vi "Configak.vi"() -> ()   [LabVIEW 2020]
uses:
  Global_Variable/A131258.vi
  Database/Global1.vi
  Global_Variable/Global.vi
  <vilib>/Utility/config.llb/NI_LVConfig.lvlib
panel:
  in  "系数":bool
  in  "产品型号":string(combo)
  in  "删除":bool
  in  "确定":bool
  in  "添加":bool
  in  "退出":bool
  in  "更新":bool
  in  "选项卡控件":enum32{"产品参数", "系统参数"}(tab)
  in  "复选框":bool
  in  "判定框范围":string[][](table)=[["°"], ["N"], ["°"], ["N"], ["°"], ["N"], ["°"], ["N"]]
  in  "工位坐标轴参数":string[][](table)=[["°"], ["N"], ["°"], ["N"], ["mm"], ["N"], ["mm"], ["N"]]
  in  "结果判定参数":string[][](table)=[["N"], ["N"], ["N"], ["N"], ["N"], ["N"], ["N"], ["N"], ["N"]]
  in  "工位滤波":T1
  in  "系统参数设置":string[][](table)=[[""], [""], [""], [""]]
  # "磨合台"
types:
  T1 = cluster{"左滤波":bool, "系数1":dbl, "右滤波":bool, "系数 2":dbl}
  T2 = enum8{"Enabled", "Disabled", "Disabled and Grayed Out"}
  T3 = typedef "NI_LVConfig.lvlib/Config Data RefNum.ctl" = refnum<k1>
  T4 = cluster{"用户编号":string, "用户名":string, "用户密码(密文)":string, "用户权限":string}
  T5 = cluster{"[0]":cluster{dbl, dbl}, "[1]":cluster{dbl, dbl}, "[2]":cluster{dbl, dbl}, "[3]":cluster{dbl, dbl}, "[4]":cluster{dbl, dbl}, "[5]":cluster{dbl, dbl}, "[6]":cluster{dbl, dbl}, "[7]":cluster{dbl, dbl}, "[8]":cluster{dbl, dbl}, "[9]":cluster{dbl, dbl}, "[10]":cluster{dbl, dbl}}
  T6 = cluster{"[0]":cluster{string, dbl, dbl}, "[1]":cluster{string, dbl, dbl}, "[2]":cluster{string, dbl, dbl}, "[3]":cluster{string, dbl, dbl}}
  T7 = cluster{"[0]":cluster{string, dbl, dbl}, "[1]":cluster{string, dbl, dbl}, "[2]":cluster{string, dbl, dbl}, "[3]":cluster{string, dbl, dbl}, "[4]":cluster{string, dbl, dbl}, "[5]":cluster{string, dbl, dbl}, "[6]":cluster{string, dbl, dbl}, "[7]":cluster{string, dbl, dbl}, "[8]":cluster{string, dbl, dbl}, "[9]":cluster{string, dbl, dbl}}
  T8 = cluster{"正向判定X值":cluster{"单位":string, "下限":dbl, "上限":dbl}, "正向判定Y值":cluster{"单位":string, "下限":dbl, "上限":dbl}, "逆向判定X值":cluster{"单位":string, "下限":dbl, "上限":dbl}, "逆向判定Y值":cluster{"单位":string, "下限":dbl, "上限":dbl}}
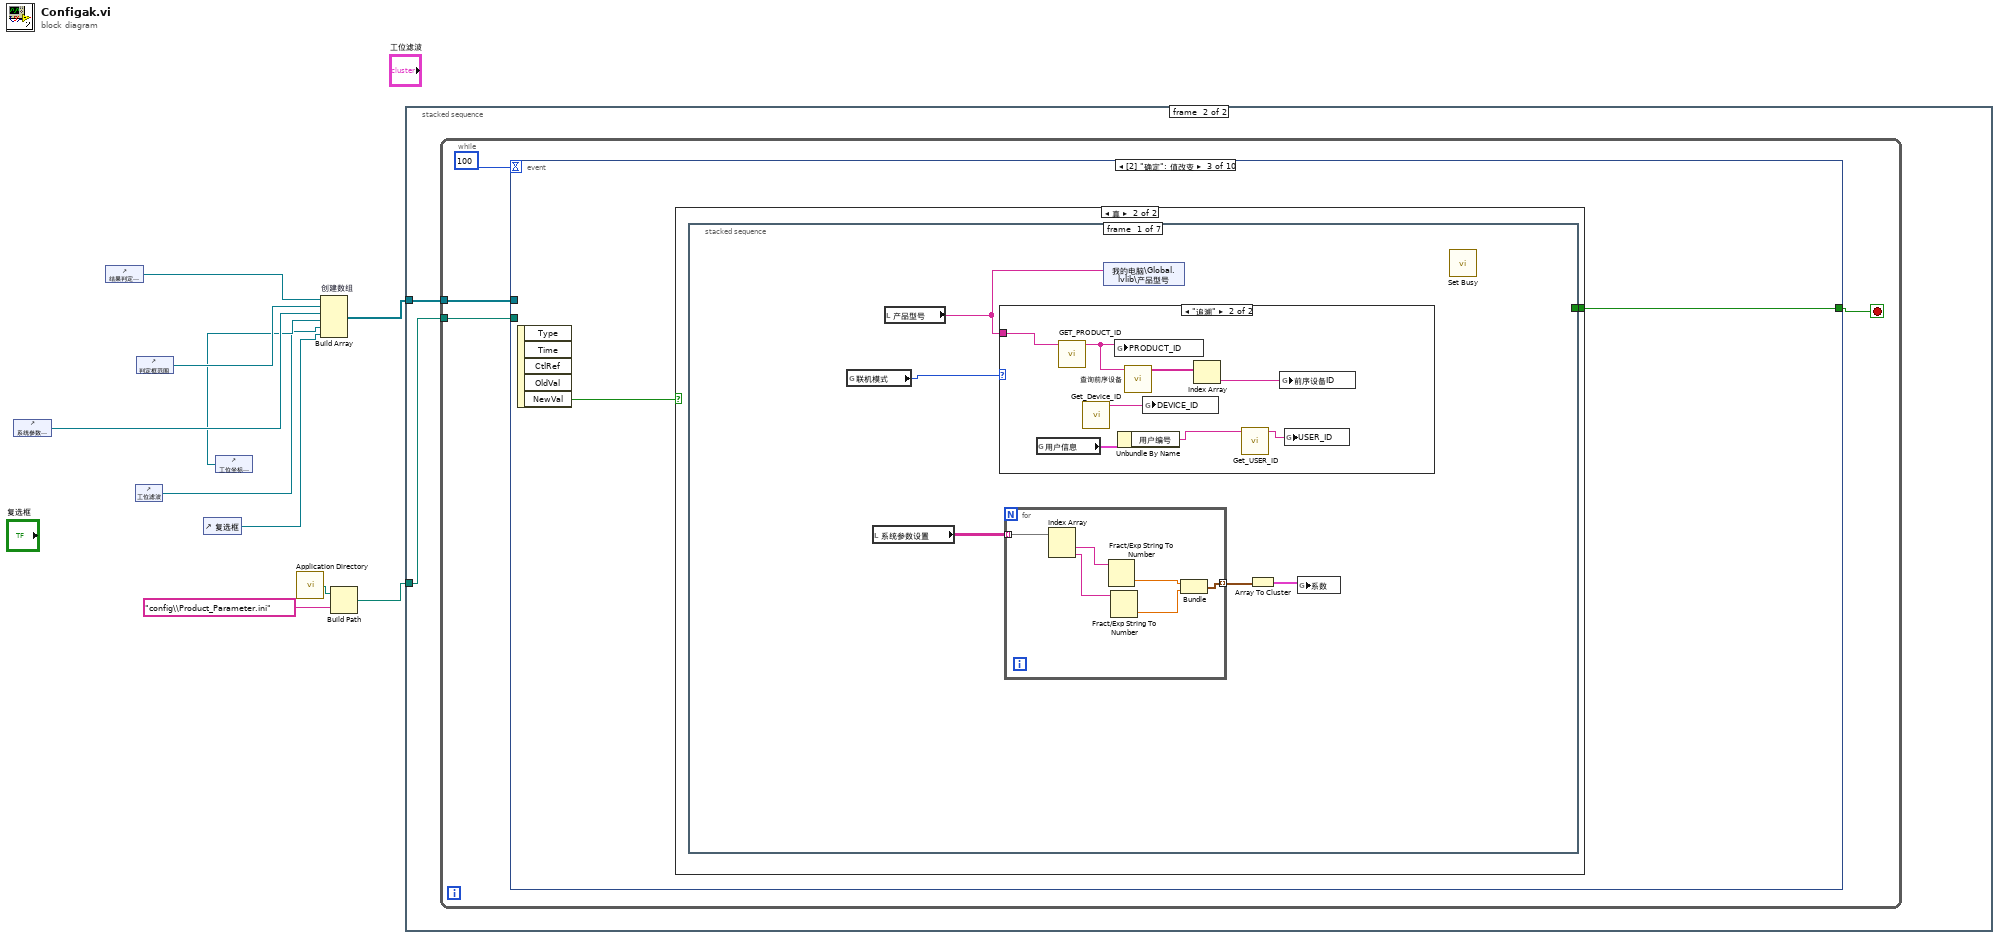
[diagram p0: block diagram]
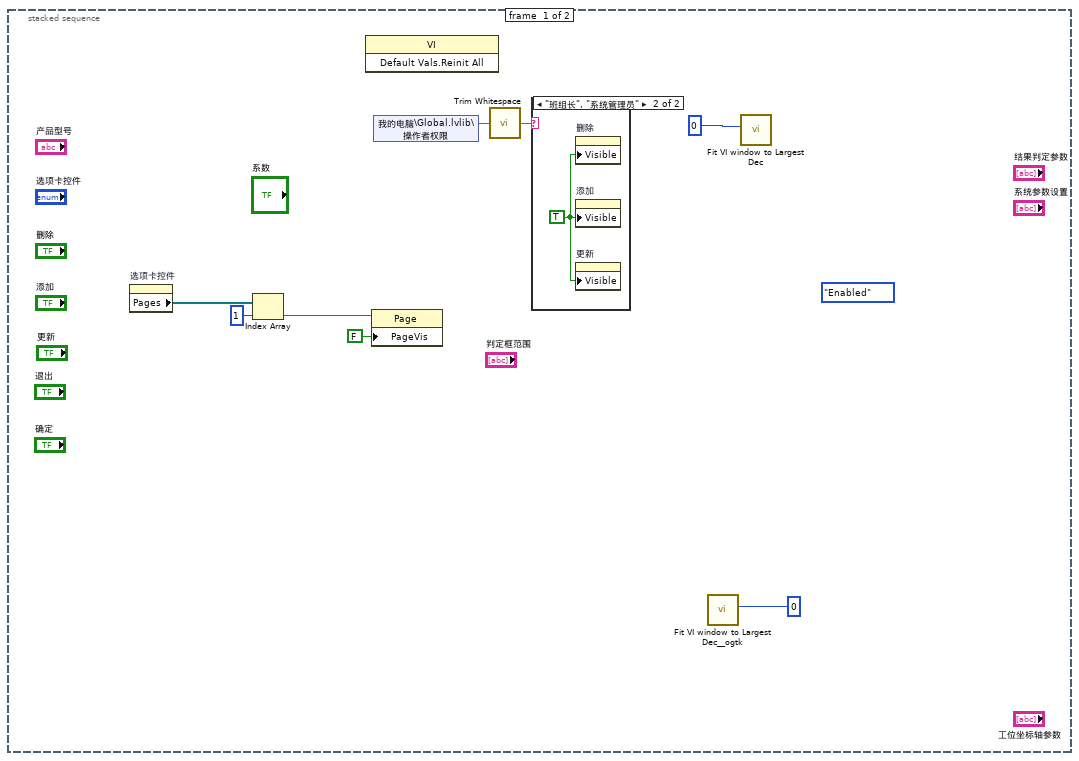
[diagram p2: hidden frame]
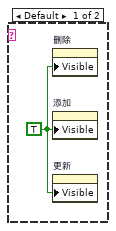
[diagram p3: hidden frame]
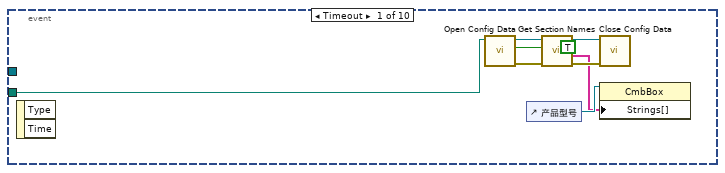
[diagram p4: hidden frame]
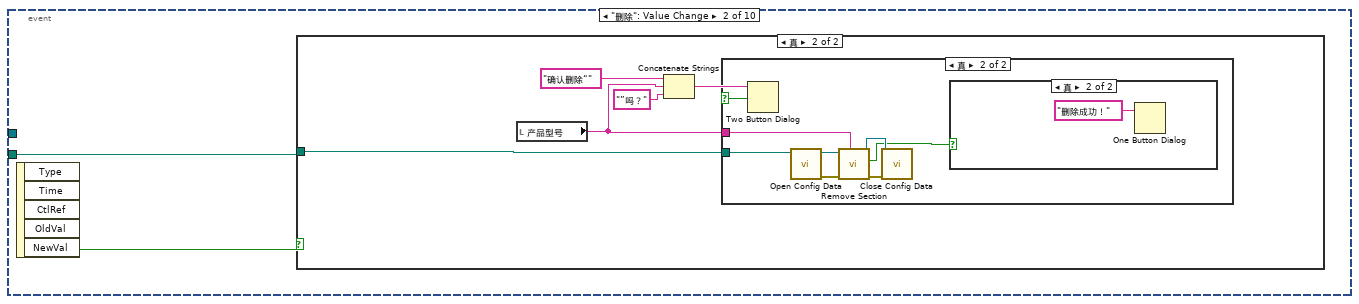
[diagram p5: hidden frame]
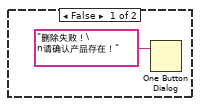
[diagram p8: hidden frame]
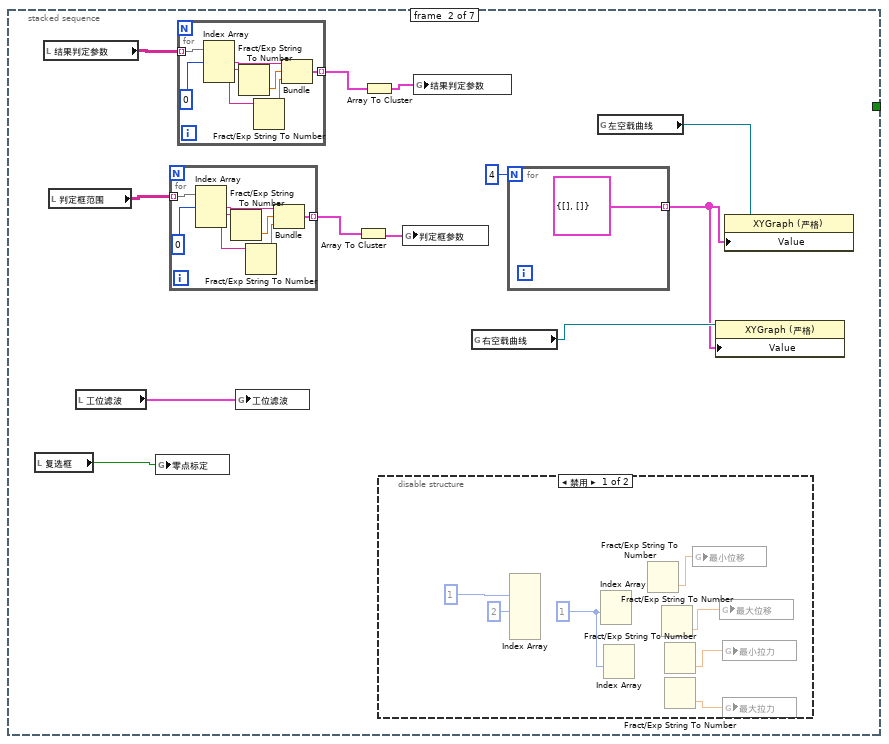
[diagram p11: hidden frame]
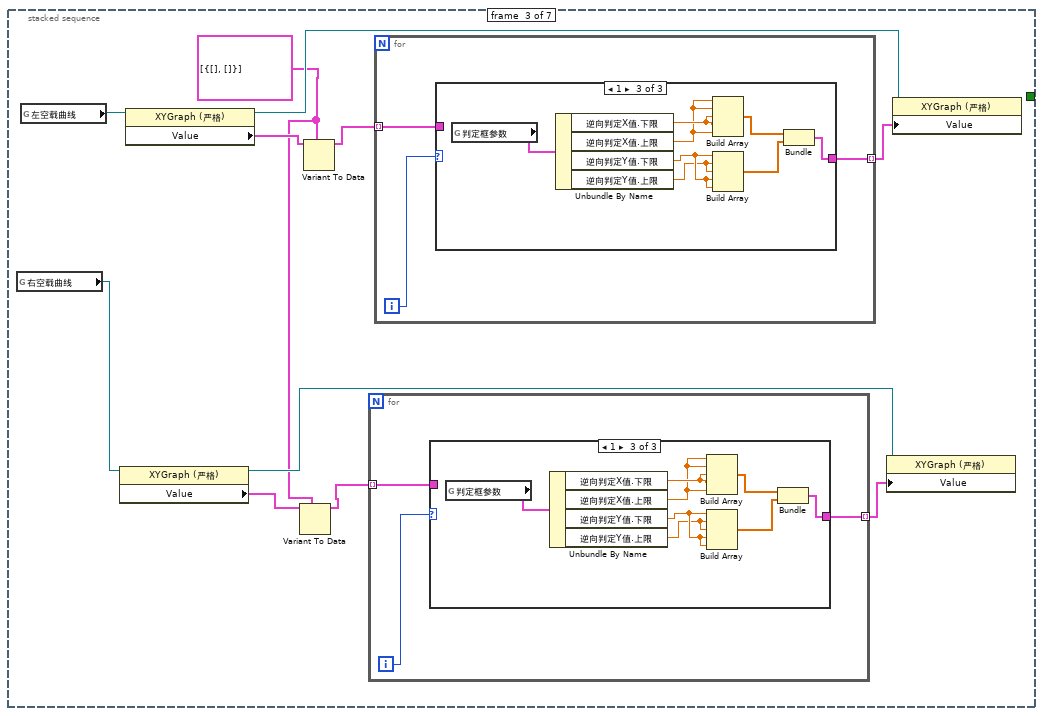
[diagram p13: hidden frame]
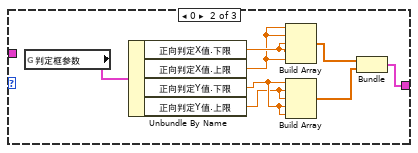
[diagram p15: hidden frame]
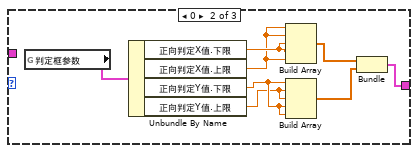
[diagram p17: hidden frame]
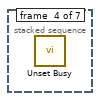
[diagram p18: hidden frame]
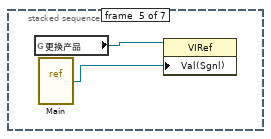
[diagram p19: hidden frame]
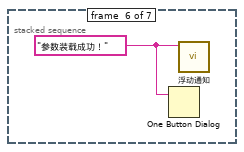
[diagram p20: hidden frame]
diagram:
  n1 = control-ref of="系统参数设置"() -> (w7:refnum<vi>)
  n2 = control-ref of="结果判定参数"() -> (w6:refnum<vi>)
  n3 = control-ref of="工位滤波"() -> (w2:refnum<vi>)
  n4 = control-ref of="判定框范围"() -> (w4:refnum<vi>)
  n5 = control-ref of="复选框"() -> (w1:refnum<vi>)
  n6 = control-ref of="工位坐标轴参数"() -> (w3:refnum<vi>)
  n7 = call <vilib>:"Application Directory.vi"() -> ("Application Directory"=w9:path)
  n8 = Build Array "创建数组"(w6, w4, w7, w3, w2, w1) -> (w10:refnum<vi>[])
  n9 = Build Path(base path=w9, name or relative path="config\\Product_Parameter.ini" ("名称或相对路径")) -> (appended path=w8:path)
  n10 = stacked-sequence {
    tunnel: w10 -> [_ w21]
    tunnel: w8 -> [_ w22]
    frame #0 {
      (unwired) T2."Enabled" ("禁用")
      n11 = property on="选项卡控件" class="TabCtl (严格)"() -> ("Pages"=w13:refnum<vi>[])  [unwired: 2 in, 2 out]
      n12 = Index Array(array=w13, index=1 ("索引")) -> (element=w14:refnum<vi>)
      n13 = invoke class="VI" method="Default Vals.Reinit All"() -> ()  [unwired: 3 in, 3 out]
      n14 = property class="Page"(reference=w14, "PageVis"=FALSE ("选项卡可见")) -> ()  [unwired: 1 in, 2 out]
      n15 = shared-variable "我的电脑\\Global.lvlib\\操作者权限"() -> (w18:string)  [unwired: 1 in, 1 out]
      n16 = call <vilib>:"Trim Whitespace.vi"("string"=w18) -> ("trimmed string"=w17:string)  [unwired: 1 in]
      n17 = case shown="\"班组长\", \"系统管理员\"" w17 {
        frame Default {
          w19 = TRUE ("可见")
          n18 = property on="删除" class="Bool (严格)"("Visible"=w19) -> ()  [unwired: 2 in, 2 out]
          n19 = property on="添加" class="Bool (严格)"("Visible"=w19) -> ()  [unwired: 2 in, 2 out]
          n20 = property on="更新" class="Bool (严格)"("Visible"=w19) -> ()  [unwired: 2 in, 2 out]
        }
        frame "班组长", "系统管理员" {
          w20 = TRUE ("可见")
          n21 = property on="删除" class="Bool (严格)"("Visible"=w20) -> ()  [unwired: 2 in, 2 out]
          n22 = property on="添加" class="Bool (严格)"("Visible"=w20) -> ()  [unwired: 2 in, 2 out]
          n23 = property on="更新" class="Bool (严格)"("Visible"=w20) -> ()  [unwired: 2 in, 2 out]
        }
      }
      n24 = call <userlib>:"Fit VI window to Largest Dec__ogtk.vi"("border spacing (2 px)"=0) -> ()  [unwired: 5 in, 2 out]
      n25 = call "Fit VI window to Largest Dec.vi"("border spacing (2 px)"=0) -> ()  [unwired: 5 in, 2 out]
    }
    frame #1 {
      n26 = while {
        tunnel: w22 -> [w26]
        tunnel: w21 -> [w23]
        stop <- w25 stop-if-true
        n27 = event shown="[2] \"确定\": 值改变" {
          selector: _ -> [_ _ _ _ _ _ _ _ _ _]
          dyn-events: _ -> [_ _ _ _ _ _ _ _ _ _]
          timeout: 100 -> [_ _ _ _ _ _ _ _ _ _]
          tunnel: w26 -> [w29 w36 _ w168 w196 _ w219 _ _ _]
          tunnel: [_ _ w52 _ _ TRUE _ _ _ TRUE] -> w25
          tunnel: w23 -> [_ _ _ w166 w194 _ w217 _ _ _]
          event Timeout {
            n28 = event-data() -> ()  [unwired: 1 in, 2 out]
            n29 = call <vilib>:"Open Config Data.vi"("create file if necessary (T)"=TRUE, "configuration file path"=w29) -> ("error out"=w31:errorcluster, "refnum"=w30:T3)  [unwired: 7 in, 1 out]
            n30 = control-ref of="产品型号"() -> (w28:refnum<vi>)
            n31 = call <vilib>:"Get Section Names.vi"("error in (no error)"=w31, "refnum"=w30) -> ("error out"=w33:errorcluster, "section names"=w27:string[], "refnum out"=w32:T3)  [unwired: 7 in]
            n32 = call <vilib>:"Close Config Data.vi"("error in (no error)"=w33, "refnum"=w32) -> ()  [unwired: 8 in, 2 out]
            n33 = property on="属性节点" class="CmbBox"(reference=w28, "Strings[]"=w27) -> ()  [unwired: 1 in, 2 out]
          }
          event "删除": Value Change {
            n34 = event-data() -> ("NewVal"=w35:bool)  [unwired: 1 in, 4 out]
            n35 = case shown="真" w35 {
              tunnel: w36 -> [_ w38]
              frame False {
              }
              frame True {
                n36 = local read "产品型号"() -> (w37:string)
                n37 = Concatenate Strings("确认删除“", w37, "”吗？") -> (w40:string)
                n38 = Two Button Dialog(message=w40) -> (T button?=w39:bool)  [unwired: 2 in]
                n39 = case shown="真" w39 {
                  tunnel: w38 -> [_ w44]
                  tunnel: w37 -> [_ w43]
                  frame False {
                  }
                  frame True {
                    n40 = call <vilib>:"Open Config Data.vi"("configuration file path"=w44) -> ("error out"=w46:errorcluster, "refnum"=w49:T3)  [unwired: 8 in, 1 out]
                    n41 = call <vilib>:"Remove Section.vi"("section"=w43, "error in (no error)"=w46, "refnum"=w49) -> ("error out"=w48:errorcluster, "section exists?"=w45:bool, "refnum out"=w47:T3)  [unwired: 6 in]
                    n42 = call <vilib>:"Close Config Data.vi"("error in (no error)"=w48, "refnum"=w47) -> ()  [unwired: 8 in, 2 out]
                    n43 = case shown="真" w45 {
                      frame False {
                        n44 = One Button Dialog(message="删除失败！\n请确认产品存在！" ("消息")) -> ()  [unwired: 1 in, 1 out]
                      }
                      frame True {
                        n45 = One Button Dialog(message="删除成功！" ("消息")) -> ()  [unwired: 1 in, 1 out]
                      }
                    }
                  }
                }
              }
            }
          }
          event "确定": Value Change {
            n46 = event-data() -> ("NewVal"=w53:bool)  [unwired: 1 in, 4 out]
            n47 = case shown="真" w53 {
              tunnel: [_ w54] -> w52
              frame False {
              }
              frame True {
                n48 = stacked-sequence {
                  tunnel: [_ _ _ _ _ _ TRUE] -> w54
                  frame #0 {
                    n49 = global read "Global1.vi" "联机模式"() -> (w58:enum16{"单机", "追溯"})
                    n50 = local read "系统参数设置"() -> (w57:string[][])
                    n51 = local read "产品型号"() -> (w59:string)
                    n52 = case shown="\"追溯\"" w58 {
                      tunnel: w59 -> [_ w73]
                      frame "单机", Default {
                      }
                      frame "追溯" {
                        n53 = global read "Global1.vi" "用户信息"() -> (w68:T4)
                        n54 = call "GET_PRODUCT_ID.vi"("PRODFUCT_NAME"=w73) -> ("PRODUCT_ID"=w72:string)  [unwired: 10 in]
                        n55 = call "Get_Device_ID.vi"() -> ("Device_ID"=w69:string)  [unwired: 10 in, 1 out]
                        n56 = global write "追溯Global.vi" "PRODUCT_ID"(w72) -> ()
                        n57 = Unbundle By Name(w68) -> ("用户编号"=w67:string)
                        n58 = call "查询前序设备.vi"("PRODUCT_ID"=w72) -> ("前序工位"=w71:string[])  [unwired: 10 in]
                        n59 = global write "追溯Global.vi" "DEVICE_ID"(w69) -> ()
                        n60 = Index Array(array=w71) -> (element=w70:string)  [unwired: 1 in]
                        n61 = call "Get_USER_ID.vi"("USER_EMPLOYEE_ID"=w67) -> ("USER_ID"=w66:string)  [unwired: 9 in, 1 out]
                        n62 = global write "追溯Global.vi" "前序设备ID"(w70) -> ()
                        n63 = global write "追溯Global.vi" "USER_ID"(w66) -> ()
                      }
                    }
                    n64 = for {
                      tunnel: w57 -> [w65] mode=indexing
                      tunnel: [w62] -> w56 mode=indexing
                      n65 = Index Array(array=w65) -> (element #1=w61:string, element #2=w60:string)  [unwired: 2 in]
                      n66 = Fract/Exp String To Number(string=w61) -> (number=w64:dbl)  [unwired: 3 in, 1 out]
                      n67 = Fract/Exp String To Number(string=w60) -> (number=w63:dbl)  [unwired: 3 in, 1 out]
                      n68 = Bundle(w64, w63) -> (w62:cluster{dbl, dbl})  [unwired: 1 in]
                    }
                    n69 = shared-variable "我的电脑\\Global.lvlib\\产品型号"(w59) -> ()  [unwired: 1 in, 1 out]
                    n70 = Array To Cluster(array=w56) -> (cluster=w55:T5)
                    n71 = global write "A131258.vi" "系数"(w55) -> ()
                    n72 = call <vilib>:"Set Busy.vi"() -> ()  [unwired: 10 in, 2 out]
                  }
                  frame #1 {
                    n73 = local read "复选框"() -> (w74:bool)
                    n74 = local read "结果判定参数"() -> (w84:string[][])
                    n75 = local read "判定框范围"() -> (w83:string[][])
                    n76 = local read "工位滤波"() -> (w75:T1)
                    n77 = global write "A131258.vi" "零点标定"(w74) -> ()
                    n78 = for {
                      tunnel: w83 -> [w97] mode=indexing
                      tunnel: [w99] -> w82 mode=indexing
                      n79 = Index Array(array=w97, index #1=0) -> (element #1=w98:string, element #2=w96:string, element #3=w95:string)  [unwired: 2 in]
                      n80 = Fract/Exp String To Number(string=w96) -> (number=w101:dbl)  [unwired: 3 in, 1 out]
                      n81 = Fract/Exp String To Number(string=w95) -> (number=w100:dbl)  [unwired: 3 in, 1 out]
                      n82 = Bundle(w98, w101, w100) -> (w99:cluster{string, dbl, dbl})  [unwired: 1 in]
                    }
                    n83 = for {
                      tunnel: w84 -> [w105] mode=indexing
                      tunnel: [w107] -> w85 mode=indexing
                      n84 = Index Array(array=w105, index #1=0) -> (element #1=w106:string, element #2=w104:string, element #3=w103:string)  [unwired: 2 in]
                      n85 = Fract/Exp String To Number(string=w104) -> (number=w109:dbl)  [unwired: 3 in, 1 out]
                      n86 = Fract/Exp String To Number(string=w103) -> (number=w108:dbl)  [unwired: 3 in, 1 out]
                      n87 = Bundle(w106, w109, w108) -> (w107:cluster{string, dbl, dbl})  [unwired: 1 in]
                    }
                    n88 = global write "A131258.vi" "工位滤波"(w75) -> ()
                    n89 = Array To Cluster(array=w82) -> (cluster=w81:T6)
                    n90 = Array To Cluster(array=w85) -> (cluster=w80:T7)
                    n91 = disable-structure shown="禁用" {
                      frame Disabled {
                        w87 = 1 ("索引")
                        n92 = Index Array(index (row) #1=1 ("索引 (行)"), index (row) #2=2 ("索引 (行)")) -> ()  [unwired: 5 in, 3 out]
                        n93 = Index Array(index #1=w87) -> ()  [unwired: 2 in, 2 out]
                        n94 = Index Array(index #1=w87) -> ()  [unwired: 2 in, 2 out]
                        n95 = Fract/Exp String To Number() -> (number=w92:dbl)  [unwired: 4 in, 1 out]
                        n96 = Fract/Exp String To Number() -> (number=w91:dbl)  [unwired: 4 in, 1 out]
                        n97 = Fract/Exp String To Number() -> (number=w90:dbl)  [unwired: 4 in, 1 out]
                        n98 = Fract/Exp String To Number() -> (number=w89:dbl)  [unwired: 4 in, 1 out]
                        n99 = global write "判定参数.vi" "最小位移"(w92) -> ()
                        n100 = global write "判定参数.vi" "最大位移"(w91) -> ()
                        n101 = global write "判定参数.vi" "最小拉力"(w90) -> ()
                        n102 = global write "判定参数.vi" "最大拉力"(w89) -> ()
                      }
                      frame Enabled {
                      }
                    }
                    n103 = global write "A131258.vi" "判定框参数"(w81) -> ()
                    n104 = global write "A131258.vi" "结果判定参数"(w80) -> ()
                    n105 = global read "A131258.vi" "右空载曲线"() -> (w77:refnum<vi>)
                    n106 = for {
                      N: 4 -> [_]
                      tunnel: [cluster{dbl[], dbl[]} {[], []}] -> w76 mode=indexing
                    }
                    n107 = global read "A131258.vi" "左空载曲线"() -> (w79:refnum<vi>)
                    n108 = property class="XYGraph (严格)"(reference=w77, "Value"=w76) -> ()  [unwired: 1 in, 2 out]
                    n109 = property class="XYGraph (严格)"(reference=w79, "Value"=w76) -> ()  [unwired: 1 in, 2 out]
                  }
                  frame #2 {
                    w113 = cluster{dbl[], dbl[]}[] [{[], []}]
                    n110 = global read "A131258.vi" "右空载曲线"() -> (w110:refnum<vi>)
                    n111 = global read "A131258.vi" "左空载曲线"() -> (w120:refnum<vi>)
                    n112 = property class="XYGraph (严格)"(reference=w110) -> (reference out=w114:refnum<vi>, "Value"=w112:cluster{"Y":dbl[], "Y":dbl[]}[])  [unwired: 1 in, 1 out]
                    n113 = property class="XYGraph (严格)"(reference=w120) -> (reference out=w119:refnum<vi>, "Value"=w117:cluster{"Y":dbl[], "Y":dbl[]}[])  [unwired: 1 in, 1 out]
                    n114 = Variant To Data(type=w113, Variant=w112) -> (data=w111:cluster{dbl[], dbl[]}[])  [unwired: 1 in, 1 out]
                    n115 = Variant To Data(type=w113, Variant=w117) -> (data=w116:cluster{dbl[], dbl[]}[])  [unwired: 1 in, 1 out]
                    n116 = for {
                      tunnel: [w122] -> w115 mode=indexing
                      tunnel: w111 -> [w121] mode=indexing
                      i -> [w123]
                      n117 = case shown="1" w123 {
                        tunnel: [w124 w130 w138] -> w122
                        tunnel: w121 -> [w124 _ _]
                        frame Default {
                        }
                        frame 0 {
                          n118 = global read "A131258.vi" "判定框参数"() -> (w129:T8)
                          n119 = Unbundle By Name(w129) -> ("正向判定X值.下限"=w128:dbl, "正向判定X值.上限"=w127:dbl, "正向判定Y值.下限"=w126:dbl, "正向判定Y值.上限"=w125:dbl)
                          n120 = Build Array(w127, w127, w128, w128, w127) -> (w132:dbl[])
                          n121 = Build Array(w126, w125, w125, w126, w126) -> (w131:dbl[])
                          n122 = Bundle(w132, w131) -> (w130:cluster{dbl[], dbl[]})  [unwired: 1 in]
                        }
                        frame 1 {
                          n123 = global read "A131258.vi" "判定框参数"() -> (w137:T8)
                          n124 = Unbundle By Name(w137) -> ("逆向判定X值.下限"=w136:dbl, "逆向判定X值.上限"=w135:dbl, "逆向判定Y值.下限"=w134:dbl, "逆向判定Y值.上限"=w133:dbl)
                          n125 = Build Array(w135, w135, w136, w136, w135) -> (w140:dbl[])
                          n126 = Build Array(w134, w133, w133, w134, w134) -> (w139:dbl[])
                          n127 = Bundle(w140, w139) -> (w138:cluster{dbl[], dbl[]})  [unwired: 1 in]
                        }
                      }
                    }
                    n128 = for {
                      tunnel: [w142] -> w118 mode=indexing
                      tunnel: w116 -> [w141] mode=indexing
                      i -> [w143]
                      n129 = case shown="1" w143 {
                        tunnel: [w144 w150 w158] -> w142
                        tunnel: w141 -> [w144 _ _]
                        frame Default {
                        }
                        frame 0 {
                          n130 = global read "A131258.vi" "判定框参数"() -> (w149:T8)
                          n131 = Unbundle By Name(w149) -> ("正向判定X值.下限"=w148:dbl, "正向判定X值.上限"=w147:dbl, "正向判定Y值.下限"=w146:dbl, "正向判定Y值.上限"=w145:dbl)
                          n132 = Build Array(w147, w147, w148, w148, w147) -> (w152:dbl[])
                          n133 = Build Array(w146, w145, w145, w146, w146) -> (w151:dbl[])
                          n134 = Bundle(w152, w151) -> (w150:cluster{dbl[], dbl[]})  [unwired: 1 in]
                        }
                        frame 1 {
                          n135 = global read "A131258.vi" "判定框参数"() -> (w157:T8)
                          n136 = Unbundle By Name(w157) -> ("逆向判定X值.下限"=w156:dbl, "逆向判定X值.上限"=w155:dbl, "逆向判定Y值.下限"=w154:dbl, "逆向判定Y值.上限"=w153:dbl)
                          n137 = Build Array(w155, w155, w156, w156, w155) -> (w160:dbl[])
                          n138 = Build Array(w154, w153, w153, w154, w154) -> (w159:dbl[])
                          n139 = Bundle(w160, w159) -> (w158:cluster{dbl[], dbl[]})  [unwired: 1 in]
                        }
                      }
                    }
                    n140 = property class="XYGraph (严格)"(reference=w114, "Value"=w115) -> ()  [unwired: 1 in, 2 out]
                    n141 = property class="XYGraph (严格)"(reference=w119, "Value"=w118) -> ()  [unwired: 1 in, 2 out]
                  }
                  frame #3 {
                    n142 = call <vilib>:"Unset Busy.vi"() -> ()  [unwired: 11 in, 1 out]
                  }
                  frame #4 {
                    n143 = global read "Global.vi" "更换产品"() -> (w162:refnum<vi>)
                    n144 = vi-ref "Main.vi"() -> (w161:refnum<vi>)
                    n145 = property class="VIRef"(reference=w162, "Val(Sgnl)"=w161) -> ()  [unwired: 1 in, 2 out]
                  }
                  frame #5 {
                    w163 = "参数装载成功！" ("消息")
                    n146 = One Button Dialog(message=w163) -> ()  [unwired: 1 in, 1 out]
                    n147 = call "浮动通知.vi"("通知内容"=w163) -> ()  [unwired: 11 in]
                  }
                  frame #6 {
                    n148 = control-ref of="本VI"() -> (w164:refnum<vi>)
                    n149 = invoke class="VI" method="FP.Close"(reference=w164) -> ()  [unwired: 2 in, 3 out]
                  }
                }
              }
            }
          }
          event "添加": Value Change {
            n150 = event-data() -> ("NewVal"=w167:bool)  [unwired: 1 in, 4 out]
            n151 = case shown="真" w167 {
              tunnel: w168 -> [_ w172]
              tunnel: w166 -> [_ w169]
              frame False {
              }
              frame True {
                n152 = call "产品添加提示：用户输入"() -> ("产品型号"=w170:string, "确定"=w171:bool)  [unwired: 17 in, 1 out]
                n153 = case shown="真" w171 {
                  tunnel: w172 -> [_ w175]
                  tunnel: w170 -> [_ w174]
                  tunnel: w169 -> [_ w173]
                  frame False {
                  }
                  frame True {
                    n154 = case shown="默认" w174 {
                      selector: w174 -> [_ w179]
                      tunnel: w175 -> [_ w181]
                      tunnel: w173 -> [_ w177]
                      frame "" {
                        n155 = One Button Dialog(message="产品名称不得为空!" ("text")) -> ()  [unwired: 1 in, 1 out]
                      }
                      frame Default {
                        n156 = property on="产品型号" class="CmbBox"() -> ("Strings[]"=w180:string[])  [unwired: 2 in, 2 out]
                        n157 = Search 1D Array(1D array=w180, element=w179) -> (index of element=w178:i32)  [unwired: 1 in]
                        n158 = case shown="-1" w178 {
                          tunnel: w181 -> [_ w185]
                          tunnel: w179 -> [_ w184]
                          tunnel: w177 -> [_ w183]
                          frame Default {
                            n159 = One Button Dialog(message="产品已存在！" ("消息")) -> ()  [unwired: 1 in, 1 out]
                          }
                          frame -1 {
                            n160 = stacked-sequence {
                              tunnel: w185 -> [w188 _]
                              tunnel: w184 -> [w187 _]
                              tunnel: w183 -> [w186 _]
                              frame #0 {
                                n161 = for {
                                tunnel: w188 -> [w192]
                                tunnel: w187 -> [w189]
                                tunnel: w186 -> [w191] mode=indexing
                                n162 = control-ref of="工位坐标轴参数"() -> ()  [unwired: 1 out]
                                n163 = call "Read_Write ParaINI File.vi"("Mode"=enum16{"Read", "Write"}."Write", "Section"=w189, "Filepath"=w192, "Ctl Refnum"=w191) -> ()  [unwired: 7 in, 1 out]
                                }
                              }
                              frame #1 {
                                n164 = One Button Dialog(message="添加成功！" ("消息")) -> ()  [unwired: 1 in, 1 out]
                              }
                            }
                          }
                        }
                      }
                    }
                  }
                }
              }
            }
          }
          event "产品型号": Value Change {
            n165 = event-data() -> ("NewVal"=w195:string)  [unwired: 1 in, 4 out]
            n166 = stacked-sequence {
              tunnel: w196 -> [_ _ w200]
              tunnel: w195 -> [_ w198 _]
              tunnel: w194 -> [_ _ w199]
              frame #0 {
                n167 = control-ref of="本VI"() -> (w197:refnum<vi>)
                n168 = invoke class="VI" method="Default Vals.Reinit All"(reference=w197) -> ()  [unwired: 2 in, 3 out]
              }
              frame #1 {
                n169 = local write "产品型号"(w198) -> ()
              }
              frame #2 {
                n170 = disable-structure shown="启用" {
                  disable-tunnel: w200 -> [w201 w209]
                  disable-tunnel: w199 -> [_ w210]
                  frame Disabled {
                    n171 = for {
                      tunnel: [w205] -> w202 mode=indexing
                      tunnel: w201 -> [w204]
                      n172 = local read "产品型号"() -> (w203:string)
                      n173 = call "Read_Write ParaINI File.vi"("Mode"=enum16{"Read", "Write"}."Read", "Section"=w203, "Filepath"=w204, "Ctl Refnum"=w205) -> ()  [unwired: 7 in, 1 out]
                    }
                  }
                  frame Enabled {
                    n174 = local read "产品型号"() -> (w211:string)
                    n175 = call <vilib>:"Set Busy.vi"() -> ("error out"=w208:errorcluster)  [unwired: 10 in, 1 out]
                    n176 = call "Read_Write INI File.vi"("Mode"=enum16{"Read", "Write"}."Read", "Section"=w211, "error in"=w208, "Filepath"=w209, "Ctl Refnum"=w210) -> ("error out"=w207:errorcluster)  [unwired: 6 in]
                    n177 = call <vilib>:"Unset Busy.vi"("error in (no error)"=w207) -> ()  [unwired: 10 in, 1 out]
                  }
                }
              }
            }
          }
          event "退出": Value Change {
            n178 = event-data() -> ()  [unwired: 1 in, 5 out]
            n179 = control-ref of="本VI"() -> (w215:refnum<vi>)
            n180 = invoke class="VI" method="FP.Close"(reference=w215) -> (reference out=w213:refnum<vi>, error out=w214:errorcluster)  [unwired: 2 in, 1 out]
            n181 = Close Reference(reference=w213, error in (no error)=w214) -> ()  [unwired: 1 out]
          }
          event "更新": Value Change {
            n182 = event-data() -> ("NewVal"=w218:bool)  [unwired: 1 in, 4 out]
            n183 = case shown="真" w218 {
              tunnel: w219 -> [_ w222]
              tunnel: w217 -> [_ w220]
              frame False {
              }
              frame True {
                n184 = for {
                  tunnel: w222 -> [w229]
                  tunnel: [w228] -> w221
                  tunnel: w220 -> [w227] mode=indexing
                  n185 = local read "产品型号"() -> (w231:string)
                  n186 = call "Read_Write ParaINI File.vi"("Mode"=enum16{"Read", "Write"}."Write", "Section"=w231, "Filepath"=w229, "Ctl Refnum"=w227) -> ("error out"=w228:errorcluster)  [unwired: 7 in]
                }
                n187 = case shown="无错误" w221 {
                  frame No Error {
                    n188 = Wait (ms)(milliseconds to wait=u32 500 ("等待时间（毫秒）")) -> ()  [unwired: 1 out]
                    n189 = One Button Dialog(message="更新成功！" ("通知内容")) -> ()  [unwired: 1 in, 1 out]
                  }
                  frame Error {
                    n190 = Wait (ms)(milliseconds to wait=u32 500 ("等待时间（毫秒）")) -> ()  [unwired: 1 out]
                    n191 = call "浮动通知.vi"("通知内容"="更新失败！") -> ()  [unwired: 11 in]
                  }
                }
              }
            }
          }
          event "系数": Mouse Enter {
            n192 = event-data() -> ()  [unwired: 1 in, 4 out]
            n193 = property on="系数" class="Bool"("Colors [4]"=cluster{u32, u32}[] [{16777216, 16777216}] ("颜色[4]")) -> ()  [unwired: 2 in, 2 out]
          }
          event "系数": Value Change {
            n194 = event-data() -> ("NewVal"=w234:bool)  [unwired: 1 in, 5 out]
            n195 = property on="选项卡控件" class="TabCtl (严格)"() -> ("Pages"=w236:refnum<vi>[])  [unwired: 2 in, 2 out]
            n196 = Index Array(array=w236, index=1 ("索引")) -> (element=w235:refnum<vi>)
            n197 = property class="Page"(reference=w235, "PageVis"=w234) -> ()  [unwired: 1 in, 2 out]
          }
          event Panel Close {
            n198 = event-data() -> ()  [unwired: 1 in, 3 out]
          }
        }
      }
    }
  }
